vi "SetAcceleration.vi"(8 "error in (no error)":errorcluster, 10 "Acceleration":dbl, 11 "ThorlabsLabJack in":refnum<class "ThorlabsLabJack.lvclass">) -> (0 "error out":errorcluster, 3 "ThorlabsLabJack out":refnum<class "ThorlabsLabJack.lvclass">)   [LabVIEW 2018, in "ThorlabsLabJack.lvlib" / "ThorlabsLabJack.lvclass"]
uses:
  ThorlabsLabJack.lvclass
  ThorlabsLabJack.lvclass/ThorlabsLabJack.ctl
  C:/Projects/LabVIEW/In-Progress/Chetan Malpure/Axis/Thorlabs LabJack/Drivers/Thorlabs.MotionControl.IntegratedStepperMotorsCLI.dll
  Drivers/Thorlabs.MotionControl.IntegratedStepperMotorsCLI.dll
  C:/Projects/LabVIEW/In-Progress/Chetan Malpure/Axis/Thorlabs LabJack/Drivers/Thorlabs.MotionControl.GenericMotorCLI.dll
  Drivers/Thorlabs.MotionControl.GenericMotorCLI.dll
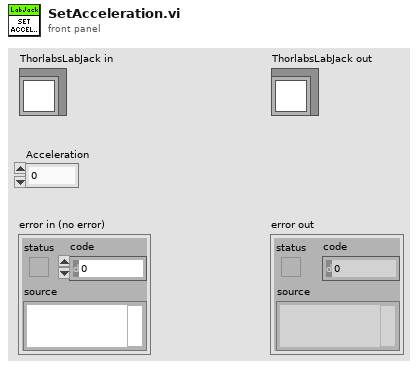
[diagram p1: front panel]
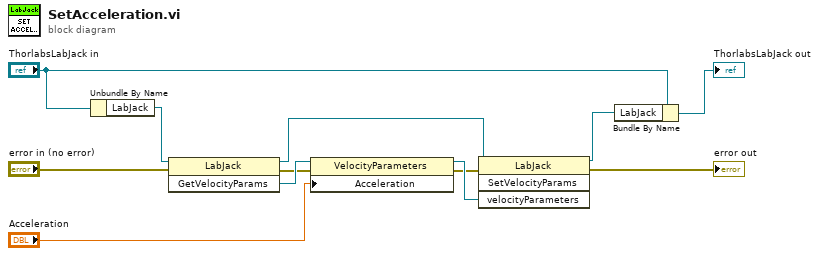
[diagram p0: block diagram]
diagram:
  n1 = Unbundle By Name("ThorlabsLabJack in") -> ("LabJack"=w8:refnum<k24>)
  n2 = invoke class="LabJack" method="GetVelocityParams"(reference=w8, error in="error in (no error)") -> (reference out=w3:refnum<k24>, error out=w5:errorcluster, "GetVelocityParams"=w6:refnum<k24>)  [unwired: 1 in]
  n3 = property class="VelocityParameters"(reference=w6, error in=w5, "Acceleration"="Acceleration") -> (reference out=w2:refnum<k24>, error out=w1:errorcluster)
  n4 = invoke class="LabJack" method="SetVelocityParams"(reference=w3, error in=w1, "velocityParameters"=w2) -> (reference out=w9:refnum<k24>, error out=→"error out":errorcluster)  [unwired: 1 in, 2 out]
  n5 = Bundle By Name(cluster="ThorlabsLabJack in", "LabJack"=w9) -> (→"ThorlabsLabJack out":refnum<class "ThorlabsLabJack.lvclass">)
